vi "Update_Software.vi"() -> ()   [LabVIEW 2010]
uses:
  Sub_vis/Update_Global.vi
panel:
  out "Incremental Update?":bool
  out "Progress":i32(slide) scale=0.0..100.0
  out "Update Location":string
  out "Current file being Saved":path
  out "No of Files updated":i32
  in  "stop":bool
  out "Current Case":string
  in  "Update from web server":bool=TRUE
  out "No of Sub vis":string[](array[string])
  out "Current Row No":i32
  out "Vis need resaving?":bool
  out "No of Source rows":i32
  out "File being copied":path
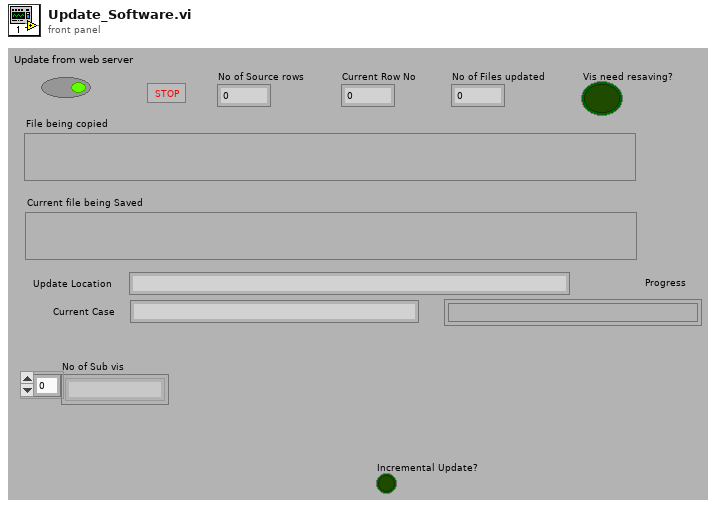
[diagram p1: front panel]
types:
  T1 = enum16{"read/write", "read-only", "write-only", "write-only (truncate)"}
  T2 = cluster{"second":i32, "minute":i32, "hour":i32, "day of month":i32, "month":i32, "year":i32, "day of week":i32, "day of year":i32, "is DST":i32}
  T3 = enum32{"existing file", "new file", "new or existing file", "existing dir", "new dir", "new or existing dir", "existing file (use LLBs)", "new file (use LLBs)", "new or existing file (use LLBs)", "new or existing file or directory (use LLBs)"}
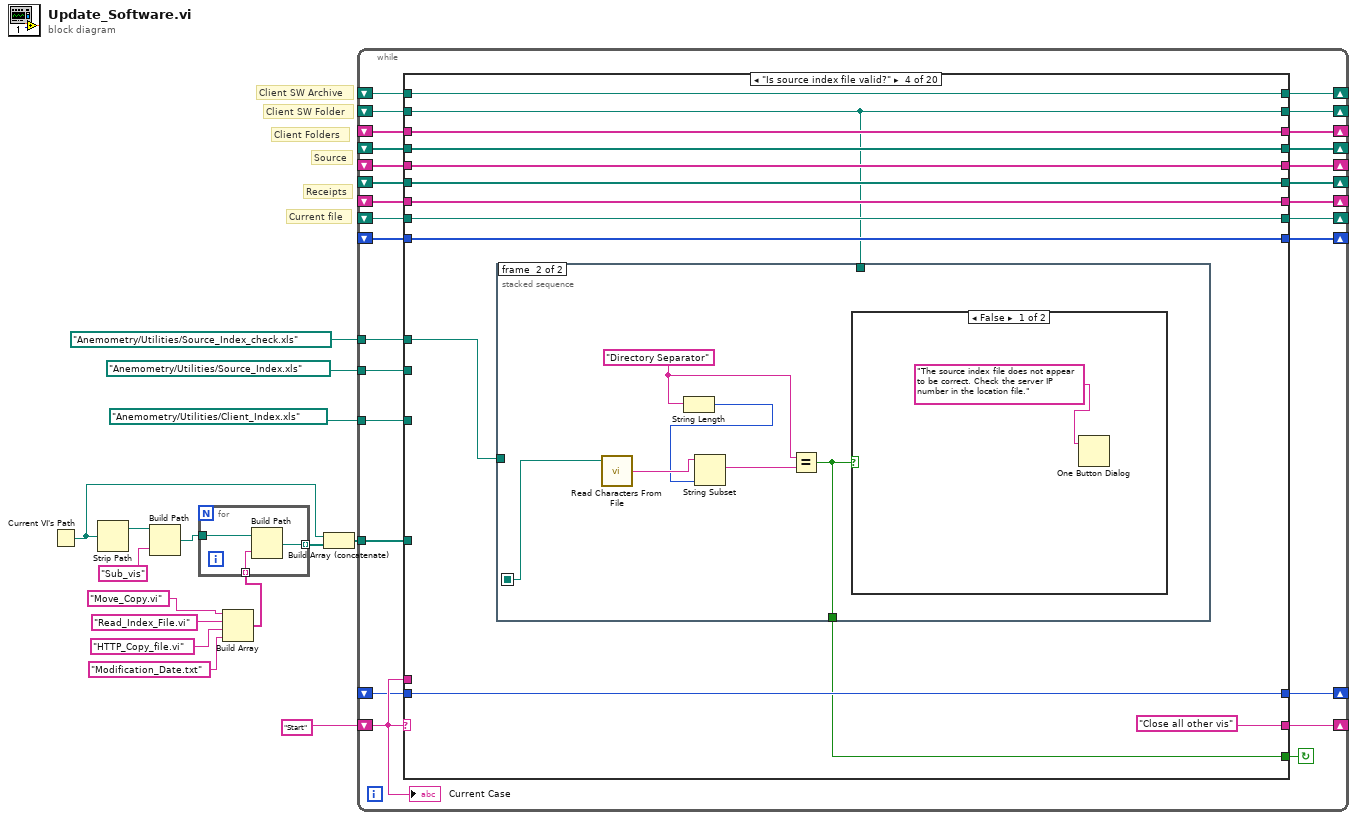
[diagram p0: block diagram]
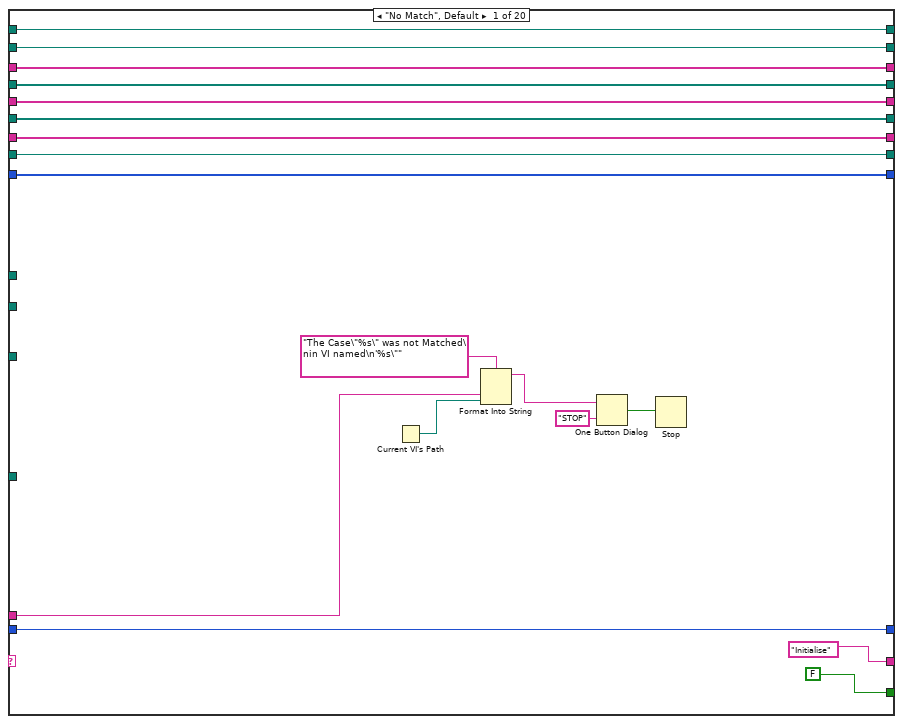
[diagram p2: hidden frame]
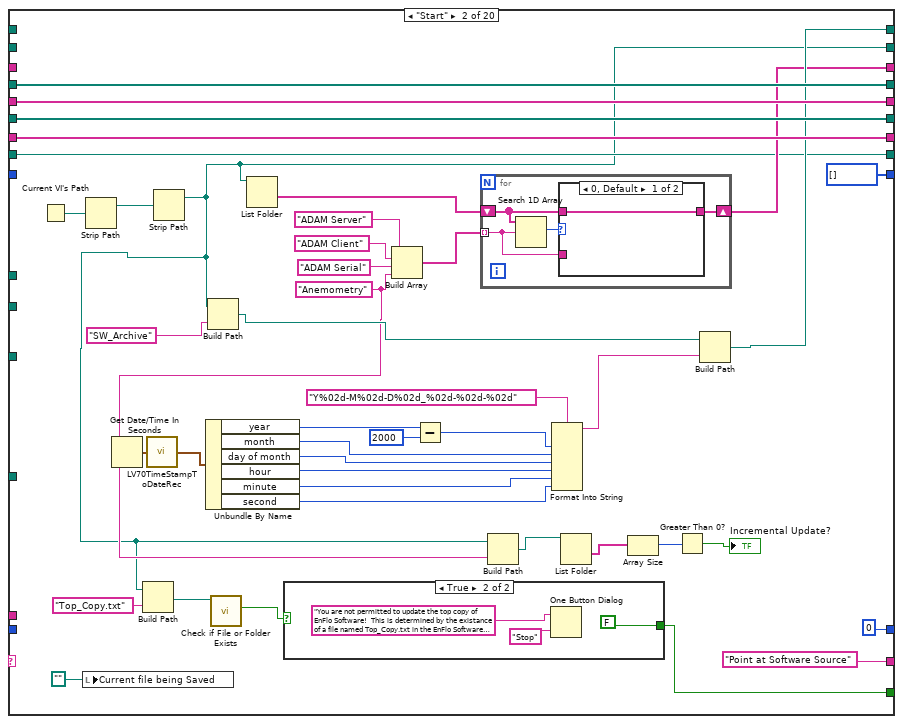
[diagram p3: hidden frame]
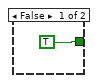
[diagram p4: hidden frame]
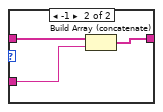
[diagram p5: hidden frame]
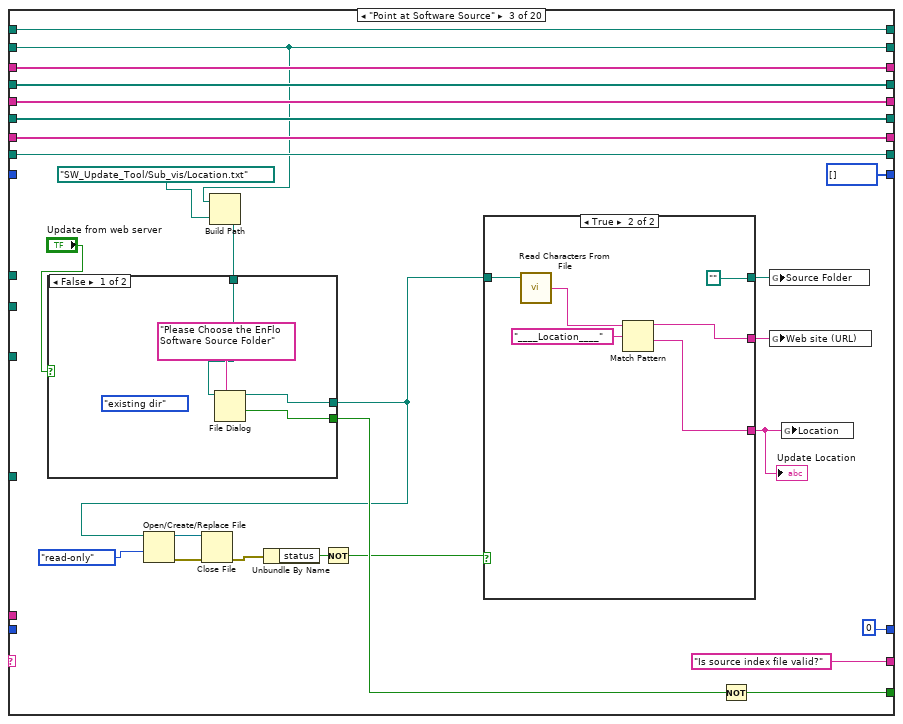
[diagram p6: hidden frame]
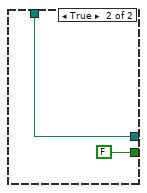
[diagram p7: hidden frame]
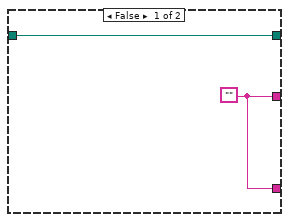
[diagram p8: hidden frame]
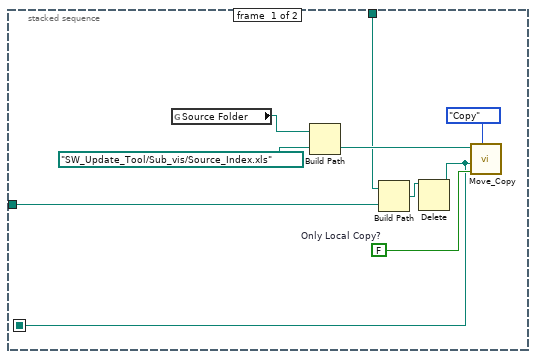
[diagram p9: hidden frame]
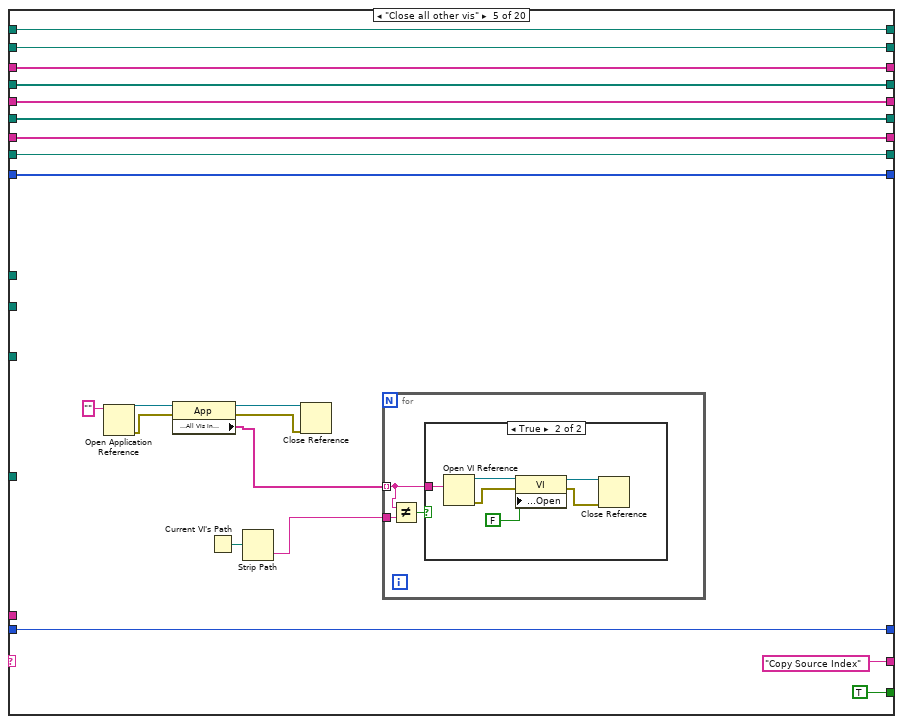
[diagram p11: hidden frame]
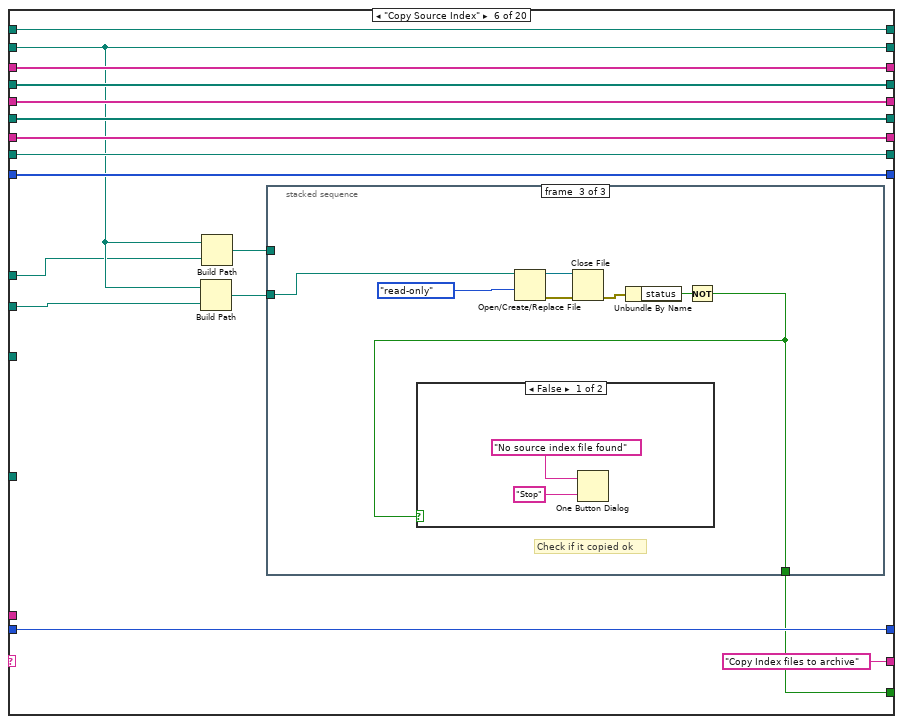
[diagram p13: hidden frame]
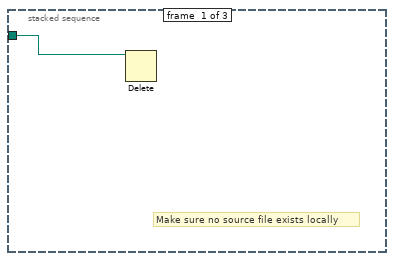
[diagram p14: hidden frame]
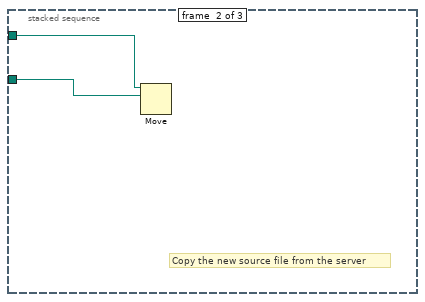
[diagram p15: hidden frame]
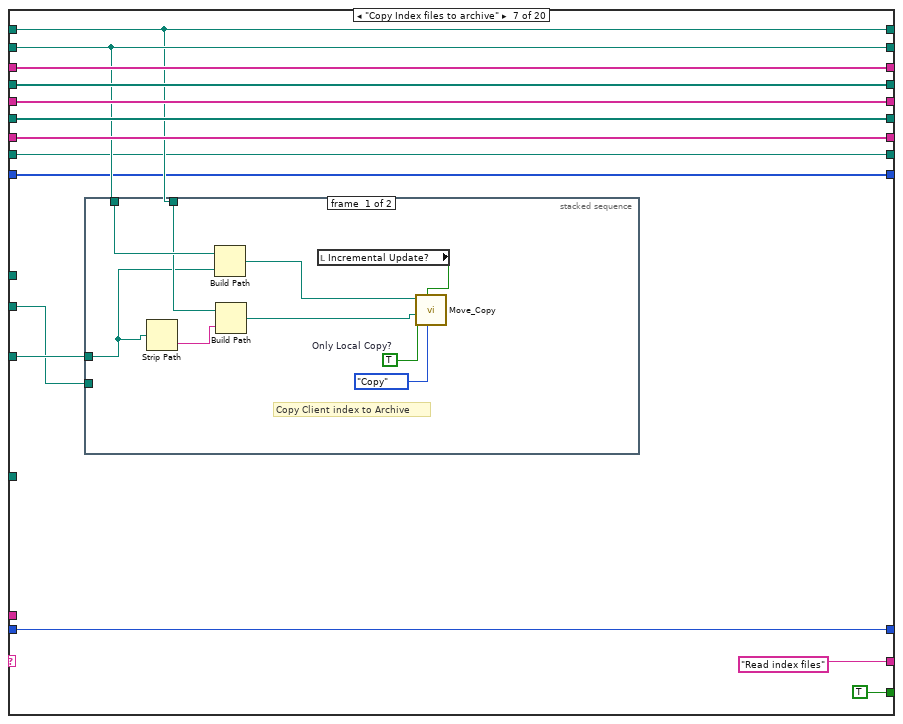
[diagram p17: hidden frame]
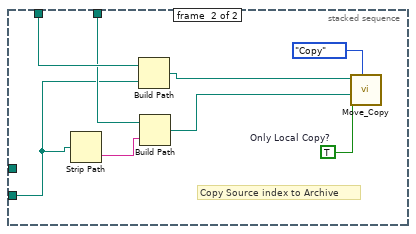
[diagram p18: hidden frame]
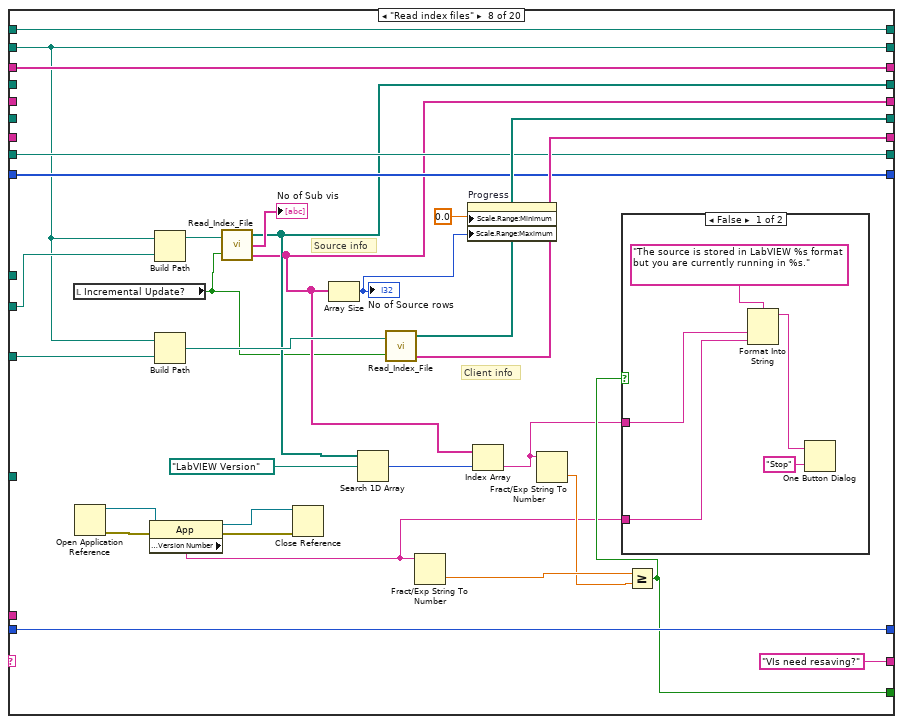
[diagram p19: hidden frame]
diagram:
  # "Current file"
  # "Receipts"
  # "Source"
  # "Client SW Archive"
  # "Client Folders"
  # "Client SW Folder"
  n1 = Current VI's Path() -> (path=w7:path)
  n2 = Strip Path(path=w7) -> (stripped path=w5:path)  [unwired: 1 out]
  n3 = Build Path(base path=w5, name or relative path="Sub_vis") -> (appended path=w3:path)
  n4 = Build Array("Move_Copy.vi", "Read_Index_File.vi", "HTTP_Copy_file.vi", "Modification_Date.txt") -> (w9:string[])
  n5 = for {
    tunnel: w3 -> [w18]
    tunnel: w9 -> [w17] mode=indexing
    tunnel: [w16] -> w8 mode=indexing
    n6 = Build Path(base path=w18, name or relative path=w17) -> (appended path=w16:path)
  }
  n7 = Build Array (concatenate)(w7, w8) -> (w6:path[])
  n8 = while {
    shift-left: "Start" -> [w43]
    shift-right: [w44] -> _
    shift-right: [w41] -> _
    shift-left: _ -> [w31]
    shift-right: [w39] -> _
    shift-left: _ -> [w40]
    shift-right: [w38] -> _
    shift-left: _ -> [w37]
    shift-right: [w35] -> _
    shift-left: _ -> [w36]
    shift-right: [w29] -> _
    shift-left: _ -> [w27]
    shift-right: [w42] -> _
    shift-left: _ -> [w32]
    shift-right: [w34] -> _
    shift-left: _ -> [w33]
    shift-right: [w30] -> _
    shift-left: _ -> [w28]
    tunnel: path "Anemometry/Utilities/Client_Index.xls" -> [w26]
    tunnel: path "Anemometry/Utilities/Source_Index.xls" -> [w25]
    shift-right: [w24] -> _
    shift-left: _ -> [w23]
    shift-right: [w21] -> _
    shift-left: _ -> [w22]
    tunnel: w6 -> [w20]
    tunnel: path "Anemometry/Utilities/Source_Index_check.xls" -> [w19]
    stop <- w45 continue-if-true
    n9 = case shown="\"Is source index file valid?\"" w43 {
      tunnel: [FALSE w65 w132 w158 TRUE ("Vis need resaving?") w221 TRUE ("Vis need resaving?") w280 TRUE TRUE TRUE TRUE TRUE TRUE w493 TRUE TRUE ("Vis need resaving?") TRUE ("Vis need resaving?") w634 FALSE] -> w45
      tunnel: ["Initialise" "Point at Software Source" "Is source index file valid?" "Close all other vis" "Copy Source Index" "Copy Index files to archive" "Read index files" "VIs need resaving?" "Valid Folder?" w364 w385 w407 w424 "Continue?" w496 "Update Receipts File" w538 "Quit LabVIEW" ("f") "Shut Update_Software" "End"] -> w44
      tunnel: w43 -> [w58 _ _ _ _ _ _ _ _ _ _ _ _ _ _ _ _ _ _ _]
      tunnel: [w55 w69 w121 w161 w187 w218 w250 w294 w338 w372 w389 w410 w432 w483 w504 w514 w552 w589 w635 w676] -> w42
      tunnel: [w54 w90 w134 w164 w199 w226 w252 w304 w340 w361 w388 w417 w433 w487 w503 w519 w558 w596 w642 w683] -> w41
      tunnel: w40 -> [w53 w103 w142 w170 w205 w230 w256 _ w336 w370 w386 w411 w430 w486 w509 w515 w554 w590 w638 w679]
      tunnel: [w53 w103 w142 w170 w205 w230 w256 w290 w336 w370 w386 w411 w430 w486 w509 w515 w554 w590 w638 w679] -> w39
      tunnel: [w52 w102 w141 w169 w204 w229 w255 w288 w326 w376 w381 w421 w436 w490 w508 w521 w561 w598 w644 w685] -> w38
      tunnel: w37 -> [w52 w102 w141 w169 w204 w229 w255 _ w326 w376 w381 w421 w436 w490 w508 w521 w561 w598 w644 w685]
      tunnel: w36 -> [w51 w101 w140 w168 w203 w228 w254 _ w335 w375 w387 w420 w435 w489 w507 w516 w560 w593 w639 w680]
      tunnel: [w51 w101 w140 w168 w203 w228 w254 w302 w335 w375 w387 w420 w435 w489 w507 w516 w560 w593 w639 w680] -> w35
      tunnel: [w50 w100 w139 w167 w202 w227 w253 w301 w334 w374 w383 w419 w434 w488 w506 w520 w559 w597 w643 w684] -> w34
      tunnel: w33 -> [w50 w100 w139 w167 w202 w227 w253 _ w334 w374 w383 w419 w434 w488 w506 w520 w559 w597 w643 w684]
      tunnel: w32 -> [w55 _ w121 w161 w187 w218 w250 w294 w338 w372 w389 w410 w432 w483 w504 w514 w552 w589 w635 w676]
      tunnel: w31 -> [w54 _ w134 w164 w199 w226 w252 w304 w340 w361 w388 w417 w433 w487 w503 w519 w558 w596 w642 w683]
      tunnel: [w49 w96 w135 w165 w200 w224 w249 w298 w341 w373 w390 w418 w429 w485 w505 w513 w541 w585 w637 w678] -> w30
      tunnel: [w47 0 0 w162 w188 w225 w251 w303 w339 w371 w382 w412 w431 w480 w500 w518 w557 w595 w641 w682] -> w29
      tunnel: w28 -> [w49 _ w135 w165 w200 w224 w249 w298 w341 w373 w390 w418 w429 w485 w505 w513 w541 w585 w637 w678]
      tunnel: w27 -> [w47 _ _ w162 w188 w225 w251 w303 w339 w371 w382 w412 w431 w480 w492 w518 w557 w595 w641 w682]
      tunnel: w26 -> [_ _ _ _ _ _ w245 w293 _ _ _ _ w427 _ _ w511 w548 _ _ _]
      tunnel: w25 -> [_ _ _ _ _ w220 w244 w296 _ _ _ _ _ _ _ _ w551 _ _ _]
      tunnel: [w48 w89 w137 w166 w201 w223 w248 w300 w337 w360 w379 w406 w426 w482 w502 w517 w556 w594 w640 w681] -> w24
      tunnel: w23 -> [w48 w89 w137 w166 w201 w223 w248 w300 w337 _ w379 w406 w426 w482 w502 w517 w556 w594 w640 w681]
      tunnel: w22 -> [w46 _ _ w163 w189 w222 w247 w299 w322 w358 w378 w403 w428 w481 w495 w512 w555 w591 w636 w677]
      tunnel: [w46 i32[] [] i32[] [] w163 w189 w222 w247 w299 w322 w358 w378 w403 w428 w479 w495 w512 w555 w591 w636 w677] -> w21
      tunnel: w20 -> [_ _ _ _ _ _ _ _ _ _ _ _ w423 _ _ _ _ _ _ _]
      tunnel: w19 -> [_ _ _ w160 _ w217 _ _ _ _ _ _ _ _ _ _ _ _ _ _]
      frame "No Match", Default {
        n10 = Current VI's Path() -> (path=w57:path)
        n11 = Format Into String(format string="The Case\"%s\" was not Matched\nin VI named\n'%s\"" ("Format String"), w58, w57) -> (resulting string=w61:string)  [unwired: 2 in, 1 out]
        n12 = One Button Dialog(message=w61, button name ("OK")="STOP") -> (true=w59:bool)
        n13 = Stop(stop? (T)=w59) -> ()
      }
      frame "Start" {
        w75 = "Anemometry"
        n14 = Current VI's Path() -> (path=w104:path)
        n15 = local write "Current file being Saved"(path "") -> ()
        n16 = Strip Path(path=w104) -> (stripped path=w99:path)  [unwired: 1 out]
        n17 = Get Date/Time In Seconds() -> (seconds since 1Jan1904=w71:timestamp)
        n18 = call <vilib>:"LV70TimeStampToDateRec.vi"("time stamp"=w71) -> ("date time rec"=w87:T2)
        n19 = Strip Path(path=w99) -> (stripped path=w69:path)  [unwired: 1 out]
        n20 = Build Path(base path=w69, name or relative path="Top_Copy.txt") -> (appended path=w67:path)
        n21 = Unbundle By Name(w87) -> ("year"=w79:i32, "month"=w83:i32, "day of month"=w84:i32, "hour"=w85:i32, "minute"=w86:i32, "second"=w76:i32)
        n22 = Build Path(base path=w69, name or relative path="SW_Archive") -> (appended path=w97:path)
        n23 = call <vilib>:"Check if File or Folder Exists.vi"("path"=w67) -> ("file or folder exists?"=w66:bool)  [unwired: 1 in, 9 out]
        n24 = List Folder(path=w69) -> (folder names=w92:string[])  [unwired: 1 in, 5 out]
        n25 = case shown="True" w66 {
          tunnel: [TRUE FALSE] -> w65
          frame False {
          }
          frame True {
            n26 = One Button Dialog(message="You are not permitted to update the top copy of EnFlo Software!  This is determined by the existance of a file named Top_Copy.txt in the EnFlo Software folder.", button name ("OK")="Stop") -> ()  [unwired: 1 out]
          }
        }
        n27 = Build Array("ADAM Server", "ADAM Client", "ADAM Serial", w75) -> (w91:string[])
        n28 = Subtract(x=w79, y=2000) -> (x-y=w81:i32)
        n29 = for {
          shift-right: [w110] -> w90
          shift-left: w92 -> [w112]
          tunnel: w91 -> [w111] mode=indexing
          n30 = Search 1D Array(1D array=w112, element=w111) -> (index of element=w113:i32)  [unwired: 1 out]
          n31 = case shown="0, Default" w113 {
            tunnel: w112 -> [w114 w117]
            tunnel: w111 -> [_ w116]
            tunnel: [w114 w115] -> w110
            frame 0, Default {
            }
            frame -1 {
              n32 = Build Array (concatenate)(w117, w116) -> (w115:string[])
            }
          }
        }
        n33 = Build Path(base path=w69, name or relative path=w75) -> (appended path=w70:path)
        n34 = Format Into String(format string="Y%02d-M%02d-D%02d_%02d-%02d-%02d", w81, w83, w84, w85, w86, w76) -> (resulting string=w78:string)  [unwired: 2 in, 1 out]
        n35 = List Folder(path=w70) -> (folder names=w74:string[])  [unwired: 1 in, 5 out]
        n36 = Array Size(array=w74) -> (size(s)=w73:i32)
        n37 = Greater Than 0?(x=w73) -> (x > 0?=→"Incremental Update?":bool)
        n38 = Build Path(base path=w97, name or relative path=w78) -> (appended path=w96:path)
      }
      frame "Point at Software Source" {
        n39 = Build Path(base path=w121, name or relative path=path "SW_Update_Tool/Sub_vis/Location.txt" ("start path")) -> (appended path=w119:path)
        n40 = case shown="False" "Update from web server" {
          tunnel: [w147 FALSE ("cancelled")] -> w133
          tunnel: [w145 w149] -> w125
          tunnel: w119 -> [w144 w149]
          frame False {
            (unwired) T3."existing dir" ("select mode (2)")
            n41 = File Dialog(7:"Please Choose the EnFlo Software Source Folder" ("prompt"), 11:w144) -> (1:w147:bool, 3:w145:path)  [unwired: 1 in, 6 out]
          }
          frame True {
          }
        }
        n42 = Open/Create/Replace File(file path (use dialog)=w125, access (0:read/write)=T1."read-only" ("open mode (0)")) -> (refnum out=w127:refnum<file>, error out=w130:errorcluster)  [unwired: 1 in, 4 out]
        n43 = Close File(refnum=w127, error in=w130) -> (error out=w129:errorcluster)  [unwired: 1 out]
        n44 = Unbundle By Name(w129) -> ("status"=w126:bool)
        n45 = Not(x=w126) -> (.not. x?=w124:bool)
        n46 = case shown="True" w124 {
          tunnel: [w151 path ""] -> w131
          tunnel: w125 -> [w151 w157]
          tunnel: [w150 w153] -> w123
          tunnel: [w150 w152] -> w122
          frame False {
            w150 = ""
          }
          frame True {
            n47 = call <vilib>:"Read Characters From File.vi"("file path (dialog if empty)"=w157) -> ("character string"=w156:string)  [unwired: 1 in, 7 out]
            n48 = Match Pattern(string=w156, regular expression="____Location____") -> (before substring=w153:string, after substring=w152:string)  [unwired: 3 out]
          }
        }
        "Update Location" <- w122
        n49 = Not(x=w133) -> (.not. x?=w132:bool)
        n50 = global write "Update_Global.vi" "Source Folder"(w131) -> ()
        n51 = global write "Update_Global.vi" "Web site (URL)"(w123) -> ()
        n52 = global write "Update_Global.vi" "Location"(w122) -> ()
      }
      frame "Is source index file valid?" {
        n53 = stacked-sequence {
          seq-local: [w171 _] -> [_ w185]
          tunnel: w161 -> [w174 _]
          tunnel: w160 -> [w173 _]
          tunnel: [_ w180] -> w158
          frame #0 {
            w176 = FALSE  # Only Local Copy?
            n54 = global read "Update_Global.vi" "Source Folder"() -> (w179:path)
            n55 = Build Path(base path=w179, name or relative path=path "SW_Update_Tool/Sub_vis/Source_Index.xls") -> (appended path=w175:path)
            n56 = Build Path(base path=w174, name or relative path=w173) -> (appended path=w172:path)
            n57 = Delete(path (use dialog)=w172) -> (deleted path=w171:path)  [unwired: 1 in, 5 out]
            n58 = call "Move_Copy.vi"("Mode"=enum16{"Move", "Copy"}."Copy", "Only Local Copy?"=w176, "target path"=w171, "source path"=w175) -> ()  [unwired: 1 in, 2 out]
          }
          frame #1 {
            w182 = "Directory Separator" ("Label for characters")
            n59 = call <vilib>:"Read Characters From File.vi"("file path (dialog if empty)"=w185) -> ("character string"=w184:string)  [unwired: 1 in, 7 out]
            n60 = String Length(string=w182) -> (length=w183:i32)
            n61 = String Subset(string=w184, length (rest)=w183) -> (substring=w181:string)  [unwired: 1 out]
            n62 = Equal?(x=w182, y=w181) -> (x = y?=w180:bool)
            n63 = case shown="False" w180 {
              frame False {
                n64 = One Button Dialog(message="The source index file does not appear to be correct. Check the server IP number in the location file.") -> ()  [unwired: 2 out]
              }
              frame True {
              }
            }
          }
        }
      }
      frame "Close all other vis" {
        n65 = Open Application Reference(11:"" ("machine name (\"\":  open local reference)")) -> (0:w197:errorcluster, 3:w198:refnum<vi>)  [unwired: 1 in, 2 out]
        n66 = property class="App"(reference=w198, error in=w197) -> (reference out=w196:refnum<vi>, error out=w195:errorcluster, "Application:All VIs In Memory"=w193:string[])
        n67 = Current VI's Path() -> (path=w192:path)
        n68 = Strip Path(path=w192) -> (name=w191:string)  [unwired: 1 out]
        n69 = Close Reference(reference=w196, error in (no error)=w195) -> ()  [unwired: 1 out]
        n70 = for {
          tunnel: w193 -> [w208] mode=indexing
          tunnel: w191 -> [w207]
          n71 = Not Equal?(x=w208, y=w207) -> (x != y?=w209:bool)
          n72 = case shown="True" w209 {
            tunnel: w208 -> [_ w215]
            frame False {
            }
            frame True {
              n73 = Open VI Reference(vi path=w215) -> (vi reference=w214:refnum<vi>, error out=w210:errorcluster)  [unwired: 1 in, 4 out]
              n74 = property class="VI"(reference=w214, error in=w210, "Front Panel Window:Open"=FALSE) -> (reference out=w212:refnum<vi>, error out=w211:errorcluster)
              n75 = Close Reference(reference=w212, error in (no error)=w211) -> ()  [unwired: 1 out]
            }
          }
        }
      }
      frame "Copy Source Index" {
        n76 = Build Path(base path=w218, name or relative path=w220) -> (appended path=w219:path)
        n77 = Build Path(base path=w218, name or relative path=w217) -> (appended path=w216:path)
        n78 = stacked-sequence {
          tunnel: w219 -> [w232 w234 w236]
          tunnel: [_ _ w235] -> w221
          tunnel: w216 -> [_ w233 _]
          frame #0 {
            # "Make sure no source file exists locally"
            n79 = Delete(path (use dialog)=w232) -> ()  [unwired: 1 in, 6 out]
          }
          frame #1 {
            # "Copy the new source file from the server"
            n80 = Move(source path=w233, 10:w234) -> ()  [unwired: 1 in, 5 out]
          }
          frame #2 {
            # "Check if it copied ok"
            n81 = Open/Create/Replace File(file path (use dialog)=w236, access (0:read/write)=T1."read-only" ("open mode (0)")) -> (refnum out=w241:refnum<file>, error out=w238:errorcluster)  [unwired: 1 in, 4 out]
            n82 = Close File(refnum=w241, error in=w238) -> (error out=w239:errorcluster)  [unwired: 1 out]
            n83 = Unbundle By Name(w239) -> ("status"=w237:bool)
            n84 = Not(x=w237) -> (.not. x?=w235:bool)
            n85 = case shown="False" w235 {
              frame False {
                n86 = One Button Dialog(message="No source index file found", button name ("OK")="Stop") -> ()  [unwired: 1 out]
              }
              frame True {
              }
            }
          }
        }
      }
      frame "Copy Index files to archive" {
        n87 = stacked-sequence {
          tunnel: w250 -> [w266 w274]
          tunnel: w249 -> [w265 w273]
          tunnel: w245 -> [w264 _]
          tunnel: w244 -> [_ w271]
          frame #0 {
            w260 = TRUE  # Only Local Copy?
            # "Copy Client index to Archive"
            n88 = Strip Path(path=w264) -> (name=w263:string)  [unwired: 1 out]
            n89 = Build Path(base path=w266, name or relative path=w264) -> (appended path=w259:path)
            n90 = Build Path(base path=w265, name or relative path=w263) -> (appended path=w261:path)
            n91 = local read "Incremental Update?"() -> (w258:bool)
            n92 = call "Move_Copy.vi"("Mode"=enum16{"Move", "Copy"}."Copy", "Send error message?"=w258, "Only Local Copy?"=w260, "target path"=w261, "source path"=w259) -> ()  [unwired: 2 out]
          }
          frame #1 {
            w269 = TRUE  # Only Local Copy?
            # "Copy Source index to Archive"
            n93 = Strip Path(path=w271) -> (name=w272:string)  [unwired: 1 out]
            n94 = Build Path(base path=w274, name or relative path=w271) -> (appended path=w268:path)
            n95 = Build Path(base path=w273, name or relative path=w272) -> (appended path=w267:path)
            n96 = call "Move_Copy.vi"("Mode"=enum16{"Move", "Copy"}."Copy", "Only Local Copy?"=w269, "target path"=w267, "source path"=w268) -> ()  [unwired: 1 in, 2 out]
          }
        }
      }
      frame "Read index files" {
        # "Source info"
        # "Client info"
        n97 = local read "Incremental Update?"() -> (w275:bool)
        n98 = Open Application Reference() -> (0:w287:errorcluster, 3:w286:refnum<vi>)  [unwired: 1 in, 3 out]
        n99 = property class="App"(reference=w286, error in=w287) -> (reference out=w285:refnum<vi>, error out=w284:errorcluster, "Application:Version Number"=w278:string)
        n100 = Build Path(base path=w294, name or relative path=w296) -> (appended path=w295:path)
        n101 = Build Path(base path=w294, name or relative path=w293) -> (appended path=w292:path)
        n102 = call "Read_Index_File.vi"("Index Filename"=w295, "Incremental Update?"=w275) -> ("Filenames"=w290:path[], "No of Sub vis"=→"No of Sub vis":string[], "Modification times"=w288:string[])
        n103 = Close Reference(reference=w285, error in (no error)=w284) -> ()  [unwired: 1 out]
        n104 = Array Size(array=w288) -> (size(s)=w276:i32)
        "No of Source rows" <- w276
        n105 = Search 1D Array(1D array=w290, element=path "LabVIEW Version" ("path")) -> (index of element=w289:i32)  [unwired: 1 out]
        n106 = call "Read_Index_File.vi"("Index Filename"=w292, "Incremental Update?"=w275) -> ("Filenames"=w302:path[], "Modification times"=w301:string[])  [unwired: 1 out]
        n107 = Fract/Exp String To Number(string=w278) -> (number=w283:dbl)  [unwired: 4 out]
        n108 = property on="Progress" class="Slide (strict)"("Scale.Range:Minimum"=0.0 ("Data Range:Minimum"), "Scale.Range:Maximum"=w276) -> ()  [unwired: 2 in, 2 out]
        n109 = Index Array(array=w288, index=w289) -> (element=w279:string)
        n110 = Fract/Exp String To Number(string=w279) -> (number=w282:dbl)  [unwired: 4 out]
        n111 = Greater Or Equal?(x=w283, y=w282) -> (x >= y?=w280:bool)
        n112 = case shown="False" w280 {
          tunnel: w279 -> [w308 _]
          tunnel: w278 -> [w307 _]
          frame False {
            n113 = Format Into String(format string="The source is stored in LabVIEW %s format but you are currently running in %s.", w308, w307) -> (resulting string=w305:string)  [unwired: 2 in, 1 out]
            n114 = One Button Dialog(message=w305, button name ("OK")="Stop") -> ()  [unwired: 1 out]
          }
          frame True {
          }
        }
      }
      frame "VIs need resaving?" {
        w316 = TRUE  # relative
        w317 = "b"
        n115 = Build Array("a", w317) -> (w313:string[])
        n116 = Array of Strings to Path(0:w313, 1:w316) -> (2:w314:path)
        n117 = Open Application Reference() -> (0:w333:errorcluster, 3:w330:refnum<vi>)  [unwired: 1 in, 3 out]
        n118 = Path To String(path=w314) -> (string=w321:string)
        n119 = property class="App"(reference=w330, error in=w333) -> (reference out=w331:refnum<vi>, error out=w332:errorcluster, "Operating System:Name"=w329:string, "Operating System:Version Number"=w328:string, "Application:Version Number"=w327:string)
        n120 = Match Pattern(string=w321, regular expression=w317) -> (offset past match=w318:i32)  [unwired: 4 out]
        n121 = Close Reference(reference=w331, error in (no error)=w332) -> ()  [unwired: 1 out]
        n122 = Subtract(x=w318, y=2) -> (x-y=w320:i32)
        n123 = String Subset(string=w321, offset (0)=w320, length (rest)=1 ("length")) -> (substring=w310:string)
        n124 = Build Array(w310, w329, w328, w327) -> (w311:string[])
        n125 = for {
          tunnel: w326 -> [w347] mode=indexing
          tunnel: w311 -> [w346] mode=indexing
          tunnel: [w345] -> w325 mode=indexing
          i -> [w344]
          n126 = case shown="2" w344 {
            tunnel: w347 -> [w350 w356]
            tunnel: w346 -> [w349 w354]
            tunnel: [w348 w351] -> w345
            frame 0, Default {
              n127 = Equal?(x=w350, y=w349) -> (x = y?=w348:bool)
            }
            frame 2 {
              w355 = "." ("regular expression")
              n128 = Match Pattern(string=w356, regular expression=w355) -> (before substring=w353:string)  [unwired: 4 out]
              n129 = Match Pattern(string=w354, regular expression=w355) -> (before substring=w352:string)  [unwired: 4 out]
              n130 = Equal?(x=w353, y=w352) -> (x = y?=w351:bool)
            }
          }
        }
        n131 = And Array Elements(Boolean array=w325) -> (logical AND=w324:bool)
        n132 = Not(x=w324) -> (.not. x?=→"Vis need resaving?":bool)
      }
      frame "Valid Folder?" {
        n133 = Increment(x=w371) -> (x+1=→"Current Row No":i32)
        n134 = Index Array(array=w370, index=w371) -> (element=w360:path)
        n135 = Path to Array of Strings(0:w360) -> (2:w369:string[])  [unwired: 1 out]
        n136 = Index Array(array=w369, index=0) -> (element=w367:string)
        n137 = Search 1D Array(1D array=w361, element=w367) -> (index of element=w366:i32)  [unwired: 1 out]
        n138 = Greater Or Equal To 0?(x=w366) -> (x >= 0?=w365:bool)
        n139 = Array Size(array=w358) -> (size(s)=→"No of Files updated":i32)
        n140 = Select(t="Get Receipt Time", s=w365, f="Continue?") -> (s? t:f=w364:string)
      }
      frame "Get Receipt Time" {
        n141 = Search 1D Array(1D array=w387, element=w379) -> (index of element=w384:i32)  [unwired: 1 out]
        n142 = case shown="0, Default" w384 {
          tunnel: [w393 w402] -> w385
          tunnel: w384 -> [w401 _]
          tunnel: w383 -> [w400 _]
          tunnel: w382 -> [w399 _]
          tunnel: w381 -> [w398 _]
          tunnel: "Update VI" -> [w394 w402]
          frame 0, Default {
            n143 = Index Array(array=w400, index=w401) -> (element=w396:string)
            n144 = Index Array(array=w398, index=w399) -> (element=w397:string)
            n145 = Equal?(x=w396, y=w397) -> (x = y?=w395:bool)
            n146 = Select(t="Does File Exist in Client?", s=w395, f=w394) -> (s? t:f=w393:string)
          }
          frame -1 {
          }
        }
      }
      frame "Does File Exist in Client?" {
        n147 = Build Path(base path=w410, name or relative path=w406) -> (appended path=w409:path)
        n148 = Open/Create/Replace File(file path (use dialog)=w409, access (0:read/write)=T1."read-only" ("open mode (0)")) -> (refnum out=w416:refnum<file>, error out=w413:errorcluster)  [unwired: 1 in, 4 out]
        n149 = Close File(refnum=w416, error in=w413) -> (error out=w414:errorcluster)  [unwired: 1 out]
        n150 = Unbundle By Name(w414) -> ("status"=w408:bool)
        n151 = Select(t="Update VI", s=w408, f="Continue?") -> (s? t:f=w407:string)
      }
      frame "Update VI" {
        n152 = Not Equal?(x=w426, y=w427) -> (x != y?=w425:bool)
        n153 = case shown="True" w425 {
          tunnel: w432 -> [_ w449]
          tunnel: w429 -> [_ w447]
          tunnel: w426 -> [_ w446]
          tunnel: ["Continue?" w441] -> w424
          tunnel: w423 -> [_ w445]
          frame False {
          }
          frame True {
            n154 = Build Path(base path=w449, name or relative path=w446) -> (appended path=w448:path)
            n155 = stacked-sequence {
              seq-local: [_ w457 _ _] -> [_ _ w464 w469]
              seq-local: [_ _ w463 _] -> [_ _ _ w470]
              tunnel: w448 -> [w455 w457 _ _]
              tunnel: w447 -> [w454 _ _ _]
              tunnel: w446 -> [w453 w461 _ _]
              tunnel: [_ w457 _ _] -> w444
              frame #0 {
                w450 = FALSE  # Send error message?
                w451 = FALSE  # Only Local Copy?
                n156 = Build Path(base path=w454, name or relative path=w453) -> (appended path=w452:path)
                n157 = call "Move_Copy.vi"("Mode"=enum16{"Move", "Copy"}."Move", "Send error message?"=w450, "Only Local Copy?"=w451, "target path"=w452, "source path"=w455) -> ()  [unwired: 2 out]
              }
              frame #1 {
                w458 = FALSE  # Only Local Copy?
                n158 = global read "Update_Global.vi" "Source Folder"() -> (w459:path)
                n159 = Build Path(base path=w459, name or relative path=w461) -> (appended path=w460:path)
                n160 = call "Move_Copy.vi"("Mode"=enum16{"Move", "Copy"}."Copy", "Only Local Copy?"=w458, "target path"=w457, "source path"=w460) -> ()  [unwired: 1 in, 2 out]
              }
              frame #2 {
                n161 = Open/Create/Replace File(file path (use dialog)=w464, access (0:read/write)=T1."read-only" ("open mode (0)")) -> (refnum out=w465:refnum<file>, error out=w468:errorcluster)  [unwired: 1 in, 4 out]
                n162 = Close File(refnum=w465, error in=w468) -> (error out=w467:errorcluster)  [unwired: 1 out]
                n163 = Unbundle By Name(w467) -> ("status"=w463:bool)
              }
              frame #3 {
                n164 = case shown="True" w470 {
                  tunnel: w469 -> [_ w472]
                  frame False {
                  }
                  frame True {
                    n165 = Strip Path(path=w472) -> (name=w471:string)  [unwired: 1 out]
                    n166 = Format Into String(format string="The file \n%s\n has not be copied from the server" ("message"), w471) -> (resulting string=w478:string)  [unwired: 2 in, 1 out]
                    n167 = Two Button Dialog(message=w478, 1:"Stop" ("button name (\"OK\")"), 2:"Continue" ("T button name (\"OK\")")) -> (T button?=w475:bool)
                    n168 = Not(x=w475) -> (.not. x?=w476:bool)
                    n169 = Stop(stop? (T)=w476) -> ()
                  }
                }
              }
            }
            n170 = Search 1D Array(1D array=w445, element=w444) -> (index of element=w443:i32)  [unwired: 1 out]
            n171 = Less Than 0?(x=w443) -> (x < 0?=w442:bool)
            n172 = Select(t="Add file to array", s=w442, f="Continue?") -> (s? t:f=w441:string)
          }
        }
        "File being copied" <- w426
      }
      frame "Add file to array" {
        n173 = Build Array (concatenate)(w481, w480) -> (w479:i32[])
      }
      frame "Continue?" {
        n174 = local read "No of Source rows"() -> (w501:i32)
        n175 = Increment(x=w492) -> (x+1=w500:i32)
        n176 = Greater?(x=w501, y=w500) -> (0:w499:bool)
        n177 = Select(t="Valid Folder?", s=w499, f="Move deleted files") -> (s? t:f=w496:string)
        n178 = Not(x="stop") -> (.not. x?=w493:bool)
        "Progress" <- w492
      }
      frame "Move deleted files" {
        n179 = for {
          tunnel: w516 -> [w525] mode=indexing
          tunnel: w515 -> [w526]
          tunnel: w514 -> [w531]
          tunnel: w513 -> [w530]
          tunnel: w511 -> [w524]
          n180 = Search 1D Array(1D array=w526, element=w525) -> (index of element=w527:i32)  [unwired: 1 out]
          n181 = Not Equal?(x=w524, y=w525) -> (x != y?=w528:bool)
          n182 = Less Than 0?(x=w527) -> (x < 0?=w529:bool)
          n183 = And(x=w529, y=w528) -> (x .and. y?=w523:bool)
          n184 = case shown="True" w523 {
            tunnel: w531 -> [_ w536]
            tunnel: w530 -> [_ w535]
            tunnel: w525 -> [_ w534]
            frame False {
            }
            frame True {
              n185 = Build Path(base path=w536, name or relative path=w534) -> (appended path=w532:path)
              n186 = Build Path(base path=w535, name or relative path=w534) -> (appended path=w533:path)
              n187 = Move(source path=w532, 10:w533) -> ()  [unwired: 1 in, 5 out]
            }
          }
        }
      }
      frame "Update Receipts File" {
        n188 = Build Path(base path=w552, name or relative path=w548) -> (appended path=w547:path)
        n189 = Build Path(base path=w552, name or relative path=w551) -> (appended path=w550:path)
        n190 = Strip Path(path=w547) -> (stripped path=w549:path)  [unwired: 1 out]
        n191 = Open Application Reference() -> (0:w543:errorcluster, 3:w544:refnum<vi>)  [unwired: 1 in, 3 out]
        n192 = property class="App"(reference=w544, error in=w543) -> ("Operating System:Name"=w542:string)  [unwired: 2 out]
        n193 = Build Path(base path=w549, name or relative path="Client_Index_orig.xls") -> (appended path=w545:path)
        n194 = stacked-sequence {
          tunnel: w547 -> [_ w564 w565 _]
          tunnel: w550 -> [_ _ w566 _]
          tunnel: w545 -> [w562 w563 _ _]
          tunnel: w542 -> [_ _ _ w568]
          tunnel: w541 -> [_ _ _ w567]
          frame #0 {
            n195 = Delete(path (use dialog)=w562) -> ()  [unwired: 1 in, 6 out]
          }
          frame #1 {
            n196 = Move(source path=w564, 10:w563) -> ()  [unwired: 1 in, 5 out]
          }
          frame #2 {
            n197 = Move(source path=w566, 10:w565) -> ()  [unwired: 1 in, 5 out]
          }
          frame #3 {
            n198 = case shown="\"Mac OS\"" w568 {
              tunnel: w567 -> [_ w574]
              frame "False", Default {
              }
              frame "Mac OS" {
                w579 = TRUE  # wait until completion? (T)
                n199 = Current VI's Path() -> (path=w577:path)
                n200 = Strip Path(path=w577) -> (stripped path=w576:path)  [unwired: 1 out]
                n201 = Strip Path(path=w576) -> (stripped path=w575:path)  [unwired: 1 out]
                n202 = Build Path(base path=w574, name or relative path="Permissions_Log.txt") -> (appended path=w572:path)
                n203 = call <vilib>:"System Exec.vi"("wait until completion? (T)"=w579, "working directory"=w575, "command line"="chmod -R 775 *") -> ("standard error"=w570:string, "standard output"=w571:string)  [unwired: 3 in, 4 out]
                n204 = Concatenate Strings(w571, w570) -> (w569:string)
                n205 = call <vilib>:"Write Characters To File.vi"("character string"=w569, "file path (dialog if empty)"=w572) -> ()  [unwired: 1 in, 3 out]
              }
            }
          }
        }
        n206 = local read "Vis need resaving?"() -> (w540:bool)
        n207 = Select(t="Save copied files", s=w540, f="Quit LabVIEW") -> (s? t:f=w538:string)
      }
      frame "Save copied files" {
        n208 = local read "No of Sub vis"() -> (w592:string[])
        n209 = Current VI's Path() -> (path=w582:path)
        n210 = for {
          tunnel: w591 -> [w630] mode=indexing
          tunnel: w592 -> [w629]
          tunnel: [w627] -> w587 mode=indexing
          n211 = Index Array(array=w629, index=w630) -> (element=w628:string)
          n212 = Fract/Exp String To Number(string=w628) -> (number=w627:dbl)  [unwired: 4 out]
        }
        n213 = local write "File being copied"(path "") -> ()
        n214 = Sort 1D Array(array=w587) -> (sorted array=w588:dbl[])
        n215 = for {
          tunnel: w588 -> [w604] mode=indexing
          shift-right: [w602] -> _
          shift-left: w587 -> [w603]
          tunnel: [w600] -> w586 mode=indexing
          tunnel: [w599] -> w581
          i -> [w599]
          w601 = nan  # new element/subarray
          n216 = Search 1D Array(1D array=w603, element=w604) -> (index of element=w600:i32)  [unwired: 1 out]
          n217 = Replace Array Subset(array=w603, new element=w601, index=w600) -> (w602:dbl[])
        }
        n218 = for {
          tunnel: w591 -> [w621]
          tunnel: w590 -> [w619]
          tunnel: w589 -> [w618]
          tunnel: w586 -> [w616] mode=indexing
          tunnel: w582 -> [w615]
          i -> [w605]
          n219 = local write "Progress"(w605) -> ()
          n220 = Index Array(array=w621, index=w616) -> (element=w620:i32)
          n221 = Index Array(array=w619, index=w620) -> (element=w617:path)
          n222 = Build Path(base path=w618, name or relative path=w617) -> (appended path=w609:path)
          n223 = Not Equal?(x=w609, y=w615) -> (x != y?=w608:bool)
          n224 = Open/Create/Replace File(file path (use dialog)=w609, access (0:read/write)=T1."read-only" ("open mode (0)")) -> (refnum out=w611:refnum<file>, error out=w614:errorcluster)  [unwired: 1 in, 4 out]
          n225 = Close File(refnum=w611, error in=w614) -> (error out=w613:errorcluster)  [unwired: 1 out]
          n226 = Unbundle By Name(w613) -> ("status"=w610:bool)
          n227 = Not(x=w610) -> (.not. x?=w607:bool)
          n228 = And(x=w608, y=w607) -> (x .and. y?=w606:bool)
          n229 = case shown="True" w606 {
            tunnel: w609 -> [_ w622]
            frame False {
            }
            frame True {
              n230 = Open VI Reference(vi path=w622) -> (vi reference=w626:refnum<vi>, error out=w625:errorcluster)  [unwired: 1 in, 4 out]
              n231 = invoke class="VI" method="Save.Instrument"(reference=w626, error in=w625, "Path to saved file"=w622, "Save a Copy"=FALSE, "Without Diagram"=FALSE) -> ()  [unwired: 1 in, 6 out]
              "Current file being Saved" <- w622
            }
          }
        }
        n232 = property on="Progress" class="Slide (strict)"("Scale.Range:Maximum"=w581) -> ()  [unwired: 2 in, 2 out]
      }
      frame "Quit LabVIEW" {
        n233 = local read "No of Files updated"() -> (w633:i32)
        n234 = Less?(x=w633, y=1) -> (x < y?=w631:bool)
        n235 = case shown="False" w631 {
          tunnel: [w646 w650] -> w634
          frame False {
            n236 = Two Button Dialog(message="Software update has successfully completed.", 1:"Quit Later" ("F button name (\"Cancel\")"), 2:"Quit Updater" ("button name (\"OK\")")) -> (T button?=w646:bool)
          }
          frame True {
            n237 = Two Button Dialog(message="There are no further updates available at the moment for EnFlo Software.", 1:"Stop" ("T button name (\"OK\")"), 2:"Relaunch EnFlo Hub" ("button name (\"OK\")")) -> (T button?=w651:bool)
            n238 = case shown="True" w651 {
              tunnel: [FALSE TRUE] -> w650
              frame False {
              }
              frame True {
                w662 = FALSE ("Wait until done")
                n239 = Current VI's Path() -> (path=w668:path)
                n240 = Strip Path(path=w668) -> (stripped path=w667:path)  [unwired: 1 out]
                n241 = Strip Path(path=w667) -> (stripped path=w666:path)  [unwired: 1 out]
                n242 = Build Path(base path=w666, name or relative path=path "Anemometry/EnFlo_Hub.vi") -> (appended path=w664:path)
                n243 = Open VI Reference(vi path=w664) -> (vi reference=w663:refnum<vi>, error out=w659:errorcluster)  [unwired: 2 in, 3 out]
                n244 = property class="VI"(reference=w663, error in=w659, "Front Panel Window:Open"=TRUE) -> (reference out=w661:refnum<vi>, error out=w660:errorcluster)
                n245 = invoke class="VI" method="Run VI"(reference=w661, error in=w660, "Wait until done"=w662, "Auto Dispose Ref"=w662) -> (reference out=w658:refnum<vi>, error out=w657:errorcluster)  [unwired: 1 in, 3 out]
                n246 = Close Reference(reference=w658, error in (no error)=w657) -> ()  [unwired: 1 out]
              }
            }
          }
        }
      }
      frame "Shut Update_Software" {
        n247 = Current VI's Path() -> (path=w673:path)
        n248 = Open VI Reference(vi path=w673) -> (vi reference=w675:refnum<vi>, error out=w674:errorcluster)  [unwired: 2 in, 3 out]
        n249 = property class="VI"(reference=w675, error in=w674, "Front Panel Window:Open"=FALSE) -> (reference out=w671:refnum<vi>, error out=w670:errorcluster)
        n250 = Close Reference(reference=w671, error in (no error)=w670) -> ()  [unwired: 1 out]
      }
    }
    "Current Case" <- w43
  }
